vi "Initialize laser step.vi"(9 "Total # data points":i32, 10 "Voltage sequence":dbl[](array[numeric])) -> (0 "error out":errorcluster, 3 "Task out":refnum<k21>)   [LabVIEW 2012]
uses:
  <vilib>/DAQmx/write.llb/DAQmx Write (Analog 1D DBL 1Chan NSamp).vi
  Channels.vi
  <vilib>/DAQmx/create/channels.llb/DAQmx Create Channel (AO-Voltage-Basic).vi
  <vilib>/DAQmx/configure/timing.llb/DAQmx Timing (Sample Clock).vi
  <vilib>/DAQmx/miscellaneous.llb/DAQmx Fill In Error Info.vi
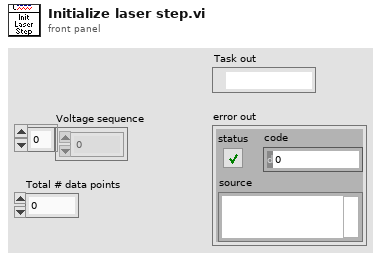
[diagram p1: front panel]
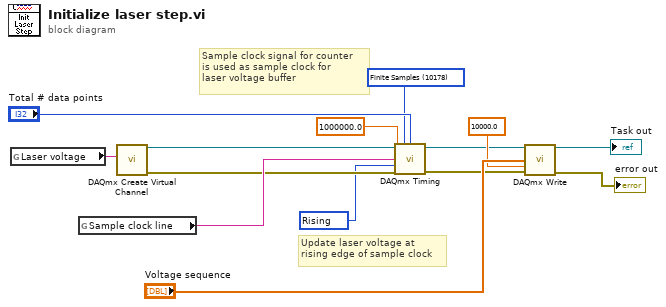
[diagram p0: block diagram]
diagram:
  w3 = 10280 items=["Rising"=10280, "Falling"=10171] ("active edge")
  w4 = 10178 items=["Finite Samples"=10178, "Continuous Samples"=10123, "Hardware Timed Single Point"=12522] ("sample mode")
  # "Update laser voltage at\nrising edge of sample clock"
  # "Sample clock signal for counter\nis used as sample clock for \nlaser voltage buffer"
  n1 = global read "Channels.vi" "Laser voltage"() -> (w1:tag)
  n2 = global read "Channels.vi" "Sample clock line"() -> (w14:tag)
  n3 = call-poly <vilib>:"DAQmx Create Virtual Channel.vi"("physical channels"=w1) -> ("task out"=w6:refnum<k21>, "error out"=w5:errorcluster)  [unwired: 13 in]
  n4 = call-poly <vilib>:"DAQmx Timing.vi"("task/channels in"=w6, "sample mode"=w4, "samples per channel"="Total # data points", "rate"=1000000.0 ("timeout"), "source"=w14, "active edge"=w3, "error in"=w5) -> ("task out"=w8:refnum<k21>, "error out"=w9:errorcluster)  [unwired: 7 in]
  n5 = call-poly <vilib>:"DAQmx Write.vi"("task/channels in"=w8, "data"="Voltage sequence", "timeout"=10000.0, "error in"=w9) -> ("task out"=→"Task out":refnum<k21>, "error out"=→"error out":errorcluster)  [unwired: 9 in, 1 out]
